vi "Tool Object.vi"(8 "error in (no error)":errorcluster, 11 "Tool Path in":refnum<class "Tool Path.lvclass">) -> (0 "error out":errorcluster, 3 "Tool Path out":refnum<class "Tool Path.lvclass">)   [LabVIEW 2019, in "Tool Path.lvclass"]
uses:
  Tool Path.lvclass
  C:/Users/Albro/Documents/GitHub/AFM-Lithography/lvsrc/Classes/Tool/Tool Object/Tool Object.lvclass
  Settings/ObjectSettings/ObjectSettings.lvclass/ObjectSettings.ctl
  Parse/PathCommands/Point.ctl
  Settings/Path Settings/Path Settings.lvclass
  C:/Users/Albro/Documents/GitHub/AFM-Lithography/lvsrc/Classes/Settings/ObjectSettings/ObjectSettings.lvclass
  Settings/ObjectSettings/ObjectSettings.lvclass
  Parse/PathCommands/PathCommands.lvclass
  Tool Object/Tool Object.lvclass
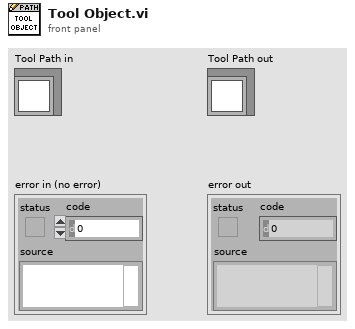
[diagram p1: front panel]
types:
  T1 = typedef "PathCommands.lvclass/Point.ctl" = cluster{"X":dbl, "Y":dbl}
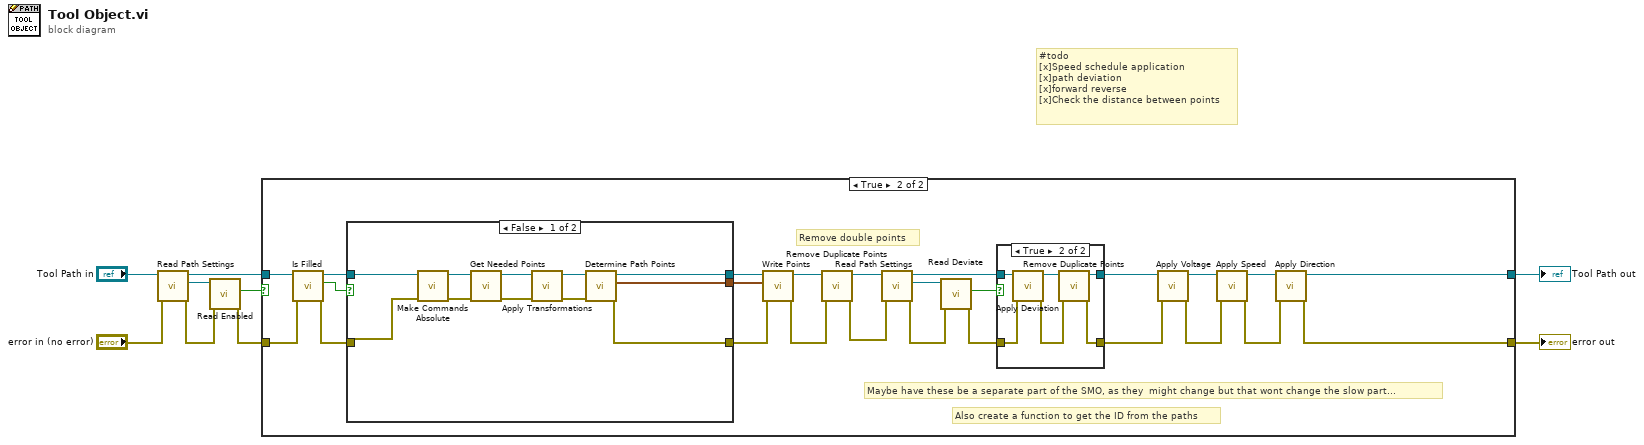
[diagram p0: block diagram]
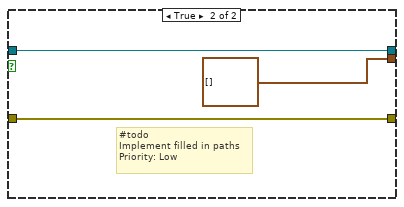
[diagram p4: hidden frame]
diagram:
  # "#todo\n[x]Speed schedule application\n[x]path deviation\n[x]forward reverse\n[x]Check the distance between points"
  n1 = call-dynamic "Read Path Settings.vi"("error in (no error)"="error in (no error)", "Tool Path in"="Tool Path in") -> ("error out"=w2:errorcluster, "Path Settings.lvclass"=w8:refnum<class "Path Settings.lvclass">, "Tool Path out"=w7:refnum<class "Tool Path.lvclass">)  [unwired: 7 in]
  n2 = call "Read Enabled.vi"("error in (no error)"=w2, "ObjectSettings in"=w8) -> ("error out"=w1:errorcluster, "Enabled"=w4:bool)  [unwired: 7 in, 1 out]
  n3 = case shown="True" w4 {
    tunnel: w7 -> [w11 w35]
    tunnel: [w11 w16] -> w6
    tunnel: w1 -> [w10 w32]
    tunnel: [w10 w17] -> w5
    frame False {
    }
    frame True {
      # "Also create a function to get the ID from the paths"
      # "Maybe have these be a separate part of the SMO, as they  might change but that wont change the slow part..."
      # "Remove double points"
      n4 = call "Is Filled.vi"("error in (no error)"=w32, "Tool Path in"=w35) -> ("error out"=w33:errorcluster, "Filled?"=w34:bool, "Tool Path out"=w36:refnum<class "Tool Path.lvclass">)  [unwired: 7 in]
      n5 = case shown="False" w34 {
        tunnel: w36 -> [w50 w58]
        tunnel: [w55 w58] -> w31
        tunnel: w33 -> [w45 w57]
        tunnel: [w54 w57] -> w30
        tunnel: [w53 T1[] [] ("Points")] -> w29
        frame False {
          n6 = call "Make Commands Absolute.vi"("error in (no error)"=w45, "Tool Path in"=w50) -> ("error out"=w48:errorcluster, "Tool Path out"=w49:refnum<class "Tool Path.lvclass">)  [unwired: 8 in]
          n7 = call-dynamic "Get Needed Points.vi"("error in (no error)"=w48, "Tool Path in"=w49) -> ("error out"=w47:errorcluster, "Tool Path out"=w46:refnum<class "Tool Path.lvclass">)  [unwired: 8 in]
          n8 = call-dynamic "Apply Transformations.vi"("error in (no error)"=w47, "Tool Path in"=w46) -> ("error out"=w51:errorcluster, "Tool Path out"=w52:refnum<class "Tool Path.lvclass">)  [unwired: 8 in]
          n9 = call-dynamic "Determine Path Points.vi"("error in (no error)"=w51, "Tool Path in"=w52) -> ("error out"=w54:errorcluster, "Points"=w53:T1[], "Tool Path out"=w55:refnum<class "Tool Path.lvclass">)  [unwired: 7 in]
        }
        frame True {
          # "#todo\nImplement filled in paths\nPriority: Low"
        }
      }
      n10 = call-dynamic "Write Points.vi"("error in (no error)"=w30, "Points"=w29, "Tool Object in"=w31) -> ("error out"=w23:errorcluster, "Tool Object out"=w28:refnum<class "Tool Path.lvclass">)  [unwired: 7 in]
      n11 = call "Remove Duplicate Points.vi"("error in (no error)"=w23, "Tool Object in"=w28) -> ("error out"=w21:errorcluster, "Tool Object out"=w14:refnum<class "Tool Path.lvclass">)  [unwired: 8 in]
      n12 = call-dynamic "Read Path Settings.vi"("error in (no error)"=w21, "Tool Path in"=w14) -> ("error out"=w25:errorcluster, "Path Settings.lvclass"=w26:refnum<class "Path Settings.lvclass">, "Tool Path out"=w27:refnum<class "Tool Path.lvclass">)  [unwired: 7 in]
      n13 = call-dynamic "Read Deviate.vi"("error in (no error)"=w25, "Path Settings in"=w26) -> ("error out"=w22:errorcluster, "Deviate"=w24:bool)  [unwired: 7 in, 1 out]
      n14 = case shown="True" w24 {
        tunnel: [w38 w42] -> w13
        tunnel: [w37 w39] -> w12
        tunnel: w27 -> [w38 w43]
        tunnel: w22 -> [w37 w44]
        frame False {
        }
        frame True {
          n15 = call-dynamic "Apply Deviation.vi"("error in (no error)"=w44, "Tool Path in"=w43) -> ("error out"=w40:errorcluster, "Tool Path out"=w41:refnum<class "Tool Path.lvclass">)  [unwired: 8 in]
          n16 = call "Remove Duplicate Points.vi"("error in (no error)"=w40, "Tool Object in"=w41) -> ("error out"=w39:errorcluster, "Tool Object out"=w42:refnum<class "Tool Path.lvclass">)  [unwired: 8 in]
        }
      }
      n17 = call-dynamic "Apply Voltage.vi"("error in (no error)"=w12, "Tool Path in"=w13) -> ("error out"=w19:errorcluster, "Tool Path out"=w20:refnum<class "Tool Path.lvclass">)  [unwired: 8 in]
      n18 = call-dynamic "Apply Speed.vi"("error in (no error)"=w19, "Tool Path in"=w20) -> ("error out"=w18:errorcluster, "Tool Path out"=w15:refnum<class "Tool Path.lvclass">)  [unwired: 8 in]
      n19 = call-dynamic "Apply Direction.vi"("error in (no error)"=w18, "Tool Path in"=w15) -> ("error out"=w17:errorcluster, "Tool Path out"=w16:refnum<class "Tool Path.lvclass">)  [unwired: 8 in]
    }
  }
  "error out" <- w5
  "Tool Path out" <- w6
